vi "AppendToOutputNew.vi"(8 "error in (no error)":errorcluster, 10 "Input String":string, 11 "String in":refnum<vi>) -> (0 "error out":errorcluster, 3 "String out":refnum<vi>)   [LabVIEW 2021]
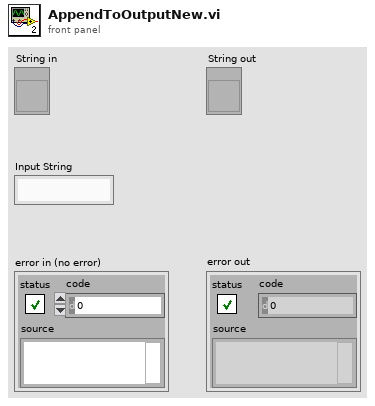
[diagram p1: front panel]
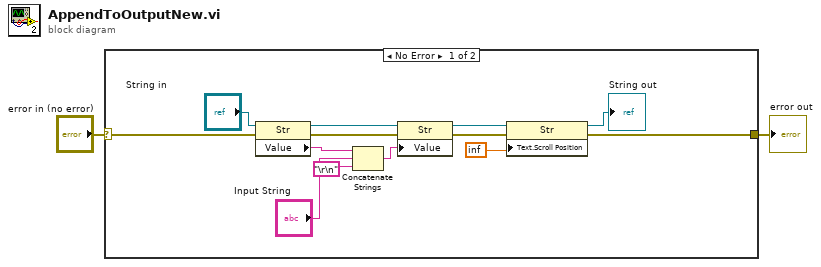
[diagram p0: block diagram]
diagram:
  n1 = case shown="No Error" "error in (no error)" {
    selector: "error in (no error)" -> [w8 w16]
    tunnel: [w3 w16] -> w1
    frame No Error {
      n2 = property on="Property Node" class="Str"(reference="String in", error in=w8) -> (reference out=w10:refnum<vi>, error out=w9:errorcluster, "Value"=w13:string)
      n3 = Concatenate Strings(w13, "Input String", "\r\n") -> (w12:string)
      n4 = property class="Str"(reference=w10, error in=w9, "Value"=w12) -> (reference out=w7:refnum<vi>, error out=w6:errorcluster)
      n5 = property class="Str"(reference=w7, error in=w6, "Text.Scroll Position"=inf) -> (reference out=→"String out":refnum<vi>, error out=w3:errorcluster)
    }
    frame Error {
    }
  }
  "error out" <- w1
